vi "RPC Method NiDAQmx CreateCIFreqChan.vi"(8 "error in (no error)":errorcluster, 11 "OOP Server in":refnum<class "NiDAQmx.lvclass">) -> (0 "error out":errorcluster, 3 "OOP Server out":refnum<class "NiDAQmx.lvclass">)   [LabVIEW 2021, in "NI DAQmx_server.lvlib" / "NiDAQmx.lvclass"]
uses:
  NiDAQmx.lvclass
  NiDAQmx.lvclass/NiDAQmx.ctl
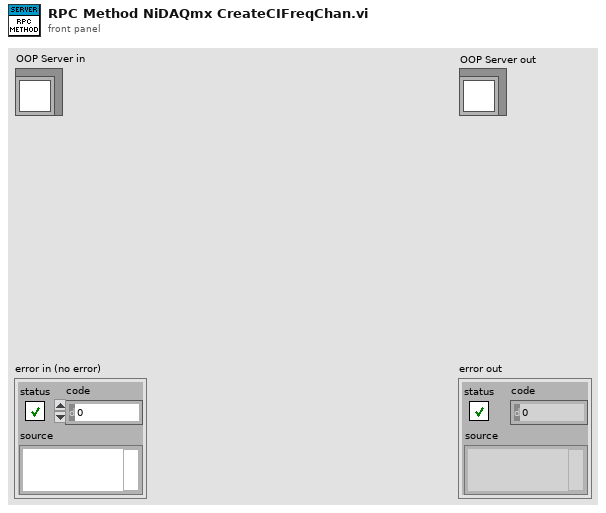
[diagram p1: front panel]
types:
  T1 = typedef "NI DAQmx_server.lvlib/NiDAQmx.lvclass/Server Internal UEs.ctl" = cluster{"NiDAQmx CreateTask Internal UE":refnum<user-event>, "NiDAQmx CreateDOChan Internal UE":refnum<user-event>, "NiDAQmx CreateCIFreqChan Internal UE":refnum<user-event>, "NiDAQmx WriteDigitalLines Internal UE":refnum<user-event>, "NiDAQmx ReadCounterScalarF64 Internal UE":refnum<user-event>, "NiDAQmx CfgImplicitTiming Internal UE":refnum<user-event>, "NiDAQmx StartTask Internal UE":refnum<user-event>, "NiDAQmx StopTask Internal UE":refnum<user-event>, "NiDAQmx ClearTask Internal UE":refnum<user-event>, "NiDAQmx GetTaskAttributeString Internal UE":refnum<user-event>, "NiDAQmx GetChanAttributeString Internal UE":refnum<user-event>, "NiDAQmx GetChanAttributeDouble Internal UE":refnum<user-event>, "NiDAQmx SetChanAttributeString Internal UE":refnum<user-event>, "NiDAQmx SetChanAttributeDouble Internal UE":refnum<user-event>}
  T2 = typedef "NI DAQmx_server.lvlib/NiDAQmx.lvclass/Server gRPC UEs.ctl" = cluster{"NiDAQmx CreateTask gRPC UE":refnum<user-event>, "NiDAQmx CreateDOChan gRPC UE":refnum<user-event>, "NiDAQmx CreateCIFreqChan gRPC UE":refnum<user-event>, "NiDAQmx WriteDigitalLines gRPC UE":refnum<user-event>, "NiDAQmx ReadCounterScalarF64 gRPC UE":refnum<user-event>, "NiDAQmx CfgImplicitTiming gRPC UE":refnum<user-event>, "NiDAQmx StartTask gRPC UE":refnum<user-event>, "NiDAQmx StopTask gRPC UE":refnum<user-event>, "NiDAQmx ClearTask gRPC UE":refnum<user-event>, "NiDAQmx GetTaskAttributeString gRPC UE":refnum<user-event>, "NiDAQmx GetChanAttributeString gRPC UE":refnum<user-event>, "NiDAQmx GetChanAttributeDouble gRPC UE":refnum<user-event>, "NiDAQmx SetChanAttributeString gRPC UE":refnum<user-event>, "NiDAQmx SetChanAttributeDouble gRPC UE":refnum<user-event>}
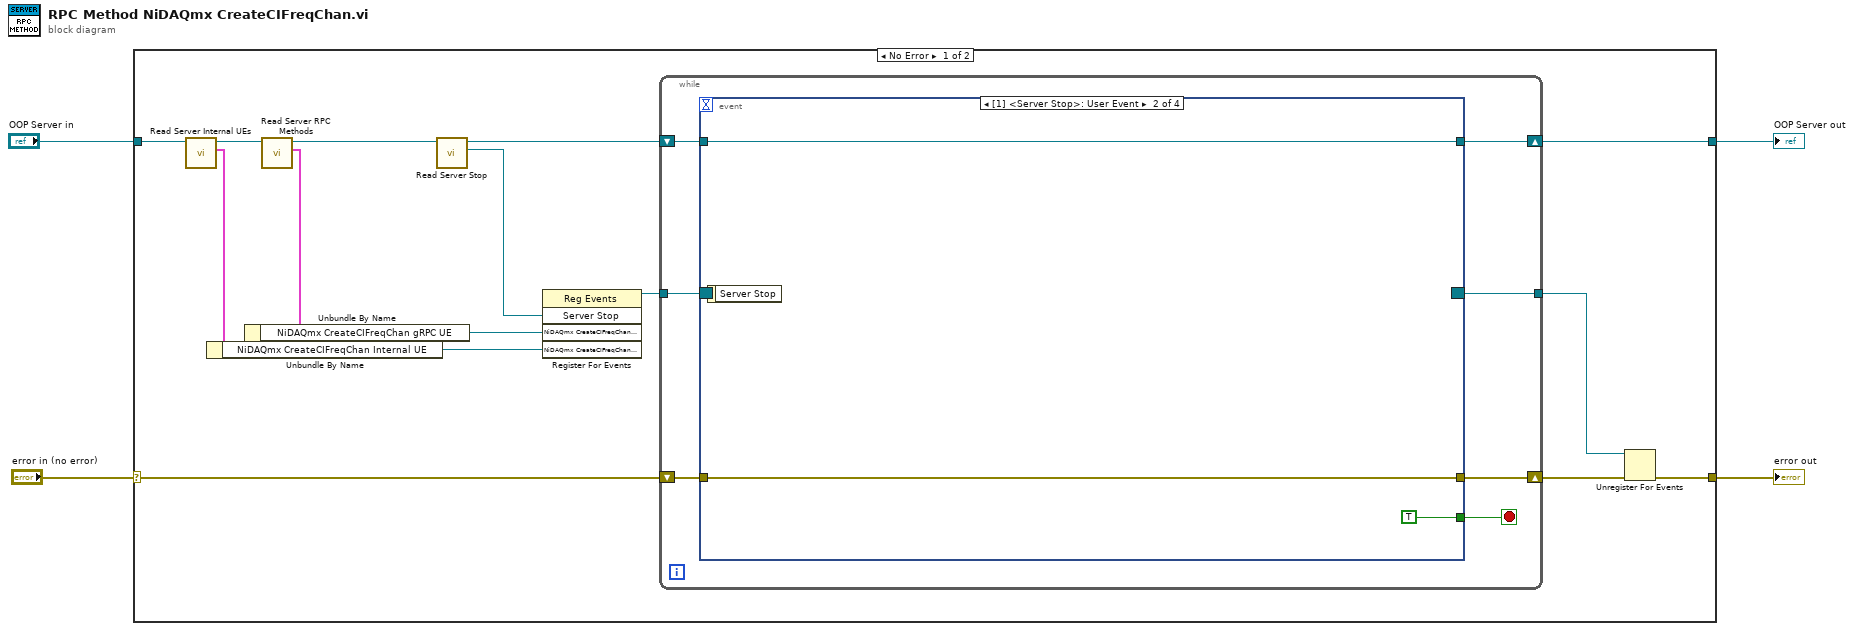
[diagram p0: block diagram]
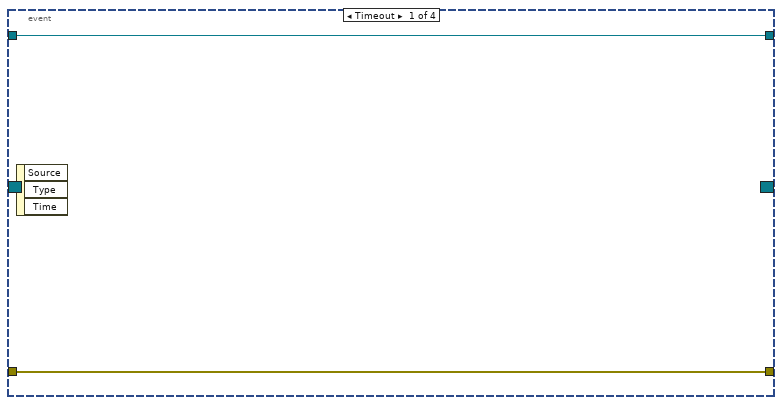
[diagram p2: hidden frame]
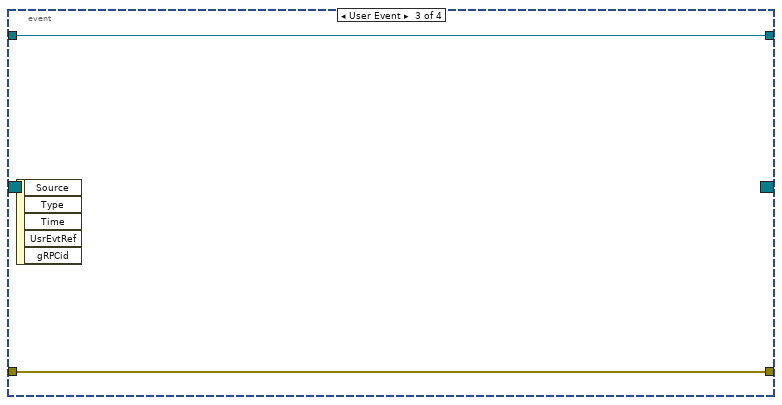
[diagram p3: hidden frame]
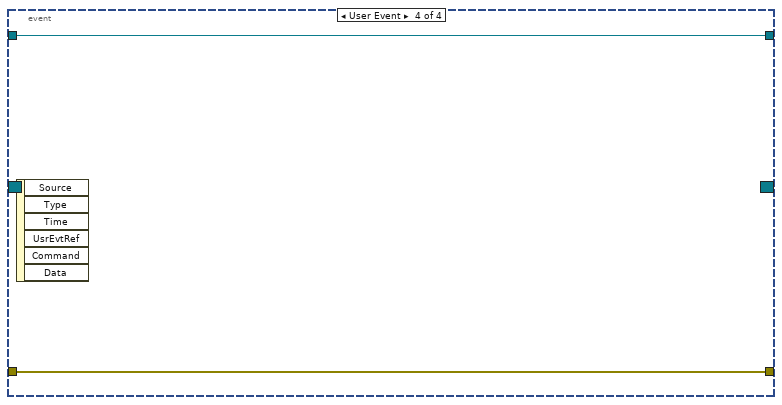
[diagram p4: hidden frame]
diagram:
  n1 = case shown="No Error" "error in (no error)" {
    selector: "error in (no error)" -> [w15 w37]
    tunnel: [w13 w37] -> w3
    tunnel: "OOP Server in" -> [w17 w36]
    tunnel: [w5 w36] -> w1
    frame No Error {
      n2 = call "Read Server Internal UEs.vi"("SignalGeneratorService in"=w17) -> ("Server Internal UEs"=w9:T1, "SignalGeneratorService out"=w16:refnum<class "NiDAQmx.lvclass">)  [unwired: 8 in, 1 out]
      n3 = Unbundle By Name ("Unbundle Internal UE")(w9) -> ("NiDAQmx CreateCIFreqChan Internal UE"=w8:refnum<user-event>)
      n4 = call "Read Server RPC Methods.vi"("SignalGeneratorService in"=w16) -> ("Server RPC Methods"=w11:T2, "SignalGeneratorService out"=w6:refnum<class "NiDAQmx.lvclass">)  [unwired: 8 in, 1 out]
      n5 = Unbundle By Name ("Unbundle gRPC UE")(w11) -> ("NiDAQmx CreateCIFreqChan gRPC UE"=w10:refnum<user-event>)
      n6 = call-dynamic "Read Server Stop.vi"("iService in"=w6) -> ("Server Stop"=w19:refnum<user-event>, "iService out"=w7:refnum<class "NiDAQmx.lvclass">)  [unwired: 8 in, 1 out]
      n7 = register-events(w19, w10, w8) -> (reference out=w18:refnum<event-registration>)  [unwired: 2 in, 1 out]
      n8 = while {
        tunnel: w18 -> [w26]
        tunnel: [w22] -> w12
        shift-right: [w23] -> w14
        shift-left: w15 -> [w24]
        shift-right: [w20] -> w5
        shift-left: w7 -> [w21]
        stop <- w25 stop-if-true
        n9 = event "RPC Method Event Structure" shown="[1] <Server Stop>: User Event" {
          selector: w26 -> [_ _ _ _]
          dyn-events: [_ _ _ _] -> w22
          timeout: _ -> [_ _ _ _]
          tunnel: [_ TRUE _ _] -> w25
          tunnel: w24 -> [w28 w30 w33 w35]
          tunnel: [w28 w30 w33 w35] -> w23
          tunnel: w21 -> [w27 w29 w32 w34]
          tunnel: [w27 w29 w32 w34] -> w20
          event Timeout {
            n10 = event-data() -> ()  [unwired: 1 in, 3 out]
          }
          event User Event {
            n11 = event-data() -> ()  [unwired: 1 in, 1 out]
          }
          event User Event {
            n12 = event-data() -> ()  [unwired: 1 in, 5 out]
          }
          event User Event {
            n13 = event-data() -> ()  [unwired: 1 in, 6 out]
          }
        }
      }
      n14 = Unregister For Events(event registration refnum=w12, error in=w14) -> (error out=w13:errorcluster)
    }
    frame Error {
    }
  }
  "error out" <- w3
  "OOP Server out" <- w1
